vi "INTEGER DATATYPES.vi"() -> ()   [LabVIEW 2019]
panel:
  in  "U64":u64
  in  "I64":i64
  in  "U32":u32
  in  "I32":i32
  in  "U16":u16
  in  "I16":i16
  in  "U8":u8
  in  "I8":i8
  # "INTEGER DATATYPES"
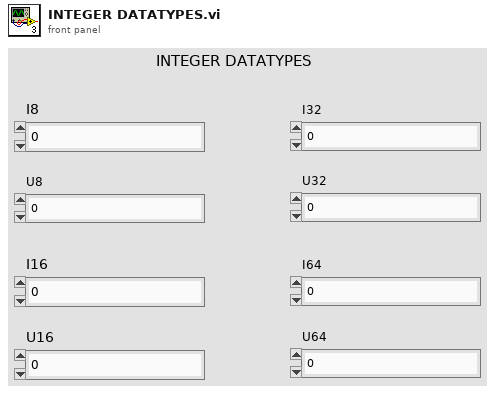
[diagram p1: front panel]
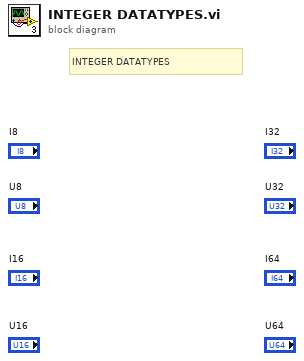
[diagram p0: block diagram]
diagram:
  # "INTEGER DATATYPES"
